vi "Mosaic.vi"(9 "Channel names":string[](array[string]), 11 "image array":u16[][][](array[numeric])) -> (3 "element out":u16[][](array[numeric]))   [LabVIEW 2023, in "Viewer.lvlib" / "Viewer.lvclass"]
uses:
  Viewer.lvclass
  Viewer.lvclass/Viewer.ctl
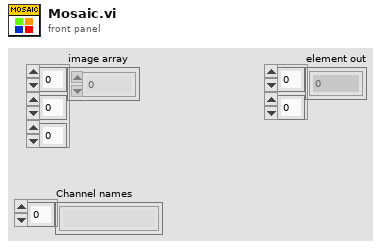
[diagram p1: front panel]
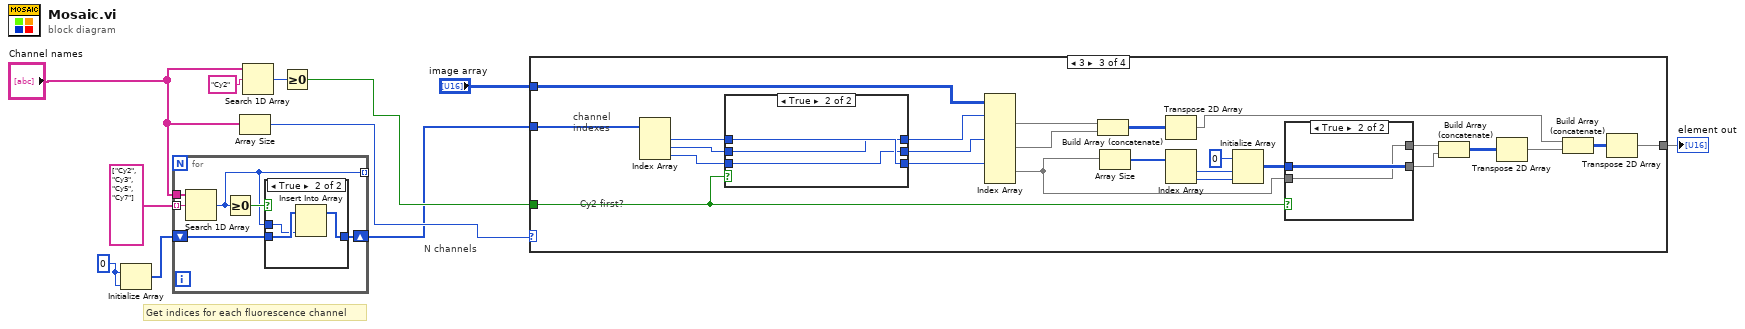
[diagram p0: block diagram]
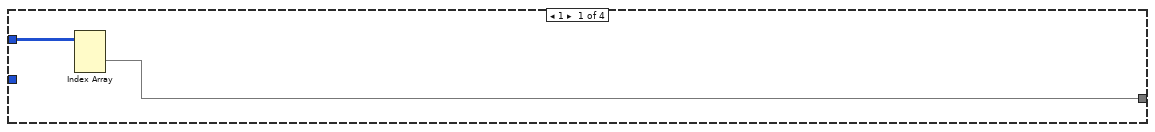
[diagram p3: hidden frame]
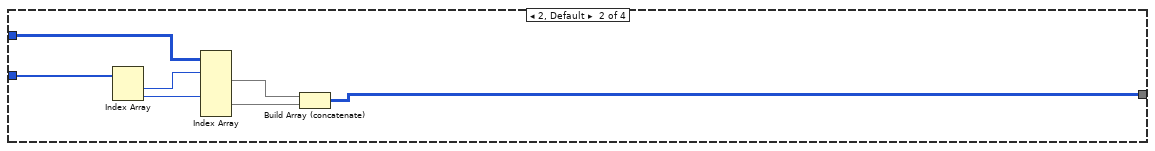
[diagram p4: hidden frame]
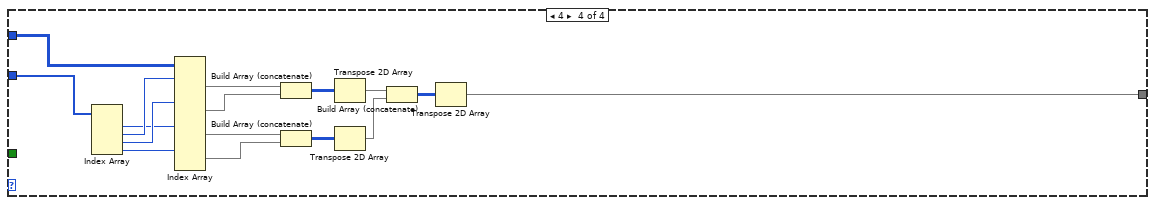
[diagram p7: hidden frame]
diagram:
  w8 = 0
  # "N channels"
  # "Get indices for each fluorescence channel"
  n1 = Initialize Array(w8, w8) -> (w7:i32[])
  n2 = for {
    tunnel: string[] ["Cy2", "Cy3", "Cy5", "Cy7"] -> [w16] mode=indexing
    tunnel: "Channel names" -> [w17]
    shift-right: [w13] -> w2
    shift-left: w7 -> [w14]
    tunnel: [w12] -> _ mode=indexing
    n3 = Search 1D Array(1D array=w17, element=w16) -> (index of element=w12:i32)  [unwired: 1 in]
    n4 = Greater Or Equal To 0?(x=w12) -> (x >= 0?=w15:bool)
    n5 = case shown="True" w15 {
      tunnel: w14 -> [w18 w21]
      tunnel: w12 -> [_ w20]
      tunnel: [w18 w19] -> w13
      frame False {
      }
      frame True {
        n6 = Insert Into Array(array=w21, new element=w20) -> (w19:i32[])  [unwired: 1 in]
      }
    }
  }
  n7 = Array Size(array="Channel names") -> (size(s)=w3:i32)
  n8 = Search 1D Array(1D array="Channel names", element="Cy2") -> (index of element=w5:i32)  [unwired: 1 in]
  n9 = Greater Or Equal To 0?(x=w5) -> (x >= 0?=w4:bool)
  n10 = case shown="3" w3 {
    tunnel: "image array" -> [w23 w30 w55 w66]
    tunnel: [w22 w29 w45 w76] -> w11
    tunnel: w2 -> [_ w28 w44 w75]
    tunnel: w4 -> [_ _ w34 _]
    frame 1 {
      n11 = Index Array(array=w23) -> (element=w22:u16[][])  [unwired: 3 in]
    }
    frame 2, Default {
      n12 = Index Array(array=w28) -> (element #1=w27:i32, element #2=w26:i32)  [unwired: 2 in]
      n13 = Index Array(array=w30, index (dim 0) #1=w27, index (dim 0) #2=w26) -> (element #1=w25:u16[][], element #2=w24:u16[][])  [unwired: 4 in]
      n14 = Build Array (concatenate)(w25, w24) -> (w29:u16[][])
    }
    frame 3 {
      # "channel\nindexes"
      # "Cy2 first?"
      n15 = Index Array(array=w44) -> (element #1=w43:i32, element #2=w41:i32, element #3=w40:i32)  [unwired: 3 in]
      n16 = case shown="True" w34 {
        tunnel: w43 -> [w62 w65]
        tunnel: [w60 w65] -> w42
        tunnel: w41 -> [w61 w64]
        tunnel: w40 -> [w60 w63]
        tunnel: [w62 w64] -> w39
        tunnel: [w61 w63] -> w38
        frame False {
        }
        frame True {
        }
      }
      n17 = Index Array(array=w55, index (dim 0) #1=w39, index (dim 0) #2=w38, index (dim 0) #3=w42) -> (element #1=w33:u16[][], element #2=w32:u16[][], element #3=w31:u16[][])  [unwired: 6 in]
      n18 = Build Array (concatenate)(w33, w32) -> (w50:u16[][])
      n19 = Array Size(array=w31) -> (size(s)=w53:i32[])
      n20 = Transpose 2D Array(2D array=w50) -> (transposed array=w47:u16[][])
      n21 = Index Array(array=w53) -> (element #1=w52:i32, element #2=w51:i32)  [unwired: 2 in]
      n22 = Initialize Array(u16 0 ("element"), w52, w51) -> (w37:u16[][])
      n23 = case shown="True" w34 {
        tunnel: w37 -> [w57 w59]
        tunnel: [w56 w59] -> w36
        tunnel: w31 -> [w56 w58]
        tunnel: [w57 w58] -> w35
        frame False {
        }
        frame True {
        }
      }
      n24 = Build Array (concatenate)(w35, w36) -> (w49:u16[][])
      n25 = Transpose 2D Array(2D array=w49) -> (transposed array=w48:u16[][])
      n26 = Build Array (concatenate)(w47, w48) -> (w46:u16[][])
      n27 = Transpose 2D Array(2D array=w46) -> (transposed array=w45:u16[][])
    }
    frame 4 {
      n28 = Index Array(array=w75) -> (element #1=w72:i32, element #2=w74:i32, element #3=w73:i32, element #4=w71:i32)  [unwired: 4 in]
      n29 = Index Array(array=w66, index (dim 0) #1=w74, index (dim 0) #2=w73, index (dim 0) #3=w72, index (dim 0) #4=w71) -> (element #1=w70:u16[][], element #2=w69:u16[][], element #3=w67:u16[][], element #4=w68:u16[][])  [unwired: 8 in]
      n30 = Build Array (concatenate)(w70, w69) -> (w81:u16[][])
      n31 = Build Array (concatenate)(w67, w68) -> (w79:u16[][])
      n32 = Transpose 2D Array(2D array=w81) -> (transposed array=w80:u16[][])
      n33 = Transpose 2D Array(2D array=w79) -> (transposed array=w78:u16[][])
      n34 = Build Array (concatenate)(w80, w78) -> (w77:u16[][])
      n35 = Transpose 2D Array(2D array=w77) -> (transposed array=w76:u16[][])
    }
  }
  "element out" <- w11
